vi "ToTable Test.vi"() -> ()   [LabVIEW 2017, in "FPGA Windows Tests.lvlib"]
doc: "Tests the 'To Table' method."
uses:
  FPGA Windows Tests.lvlib
  <vilib>/NI/Module Execution Interface/Engine Configuration/engine configuration.lvclass
  editor node/FPGA Module editor node.lvclass
  <vilib>/NI/Tag Bus/tag/tag descriptor.lvclass
  <vilib>/NI/Tag Bus/tag/Data Type.ctl
  <vilib>/NI/Tag Bus/tag/tag descriptor.lvclass/tag descriptor.ctl
  <vilib>/NI/Configuration Framework/serializable configuration/NISE_CEF_serializable configuration.lvclass/NISE_CEF_serializable configuration.ctl
  module/configuration/FPGA Module configuration.lvclass
  C:/Program Files (x86)/National Instruments/LabVIEW 2017/vi.lib/NI/Configuration Framework/serializable configuration/NISE_CEF_serializable configuration.lvclass
  <vilib>/Utility/LVClass/Get LV Class Name.vi
  <vilib>/NI/Configuration Framework/error generator/NISE_error generator.vi
  <vilib>/NI/Configuration Framework/serializable configuration/NISE_CEF_serializable configuration.lvclass
panel:
  out "error out":errorcluster
  out "table":string[][](array[string])
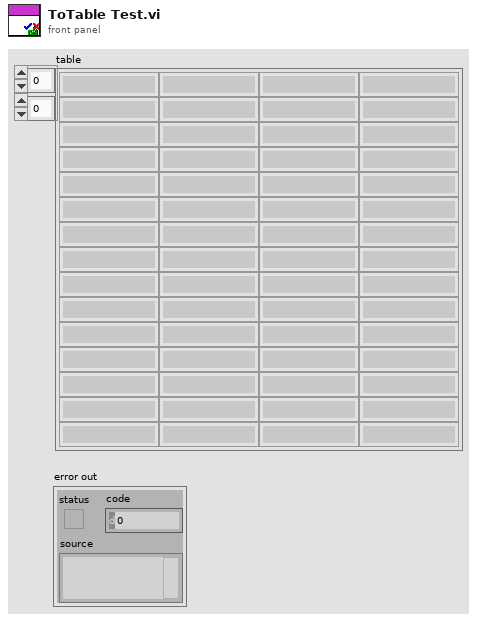
[diagram p1: front panel]
types:
  T1 = typedef "tag bus.lvlib/tag descriptor.lvclass/Data Type.ctl" = enum16{"Double", "Single", "I64", "I32", "I16", "I8", "U64", "U32", "U16", "U8", "Boolean", "String", "Array of Double", "Array of Single", "Array of I64", "Array of I32", "Array of I16", "Array of I8", "Array of U64", "Array of U32", "Array of U16", "Array of U8", "Array of Boolean", "Array of String"}
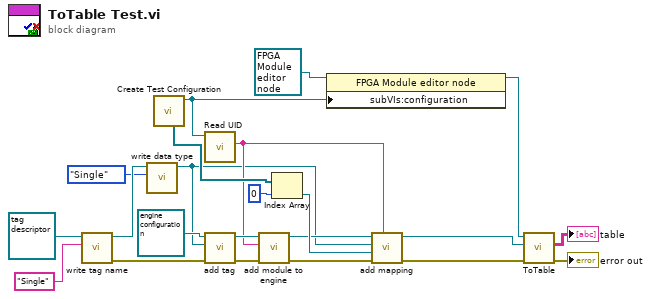
[diagram p0: block diagram]
diagram:
  n1 = call <vilib>:"write tag name.vi"("name"="Single", "system tag in"=refnum<class "tag descriptor.lvclass"> refnum ("tag descriptor")) -> ("error out"=w4:errorcluster, "system tag out"=w3:refnum<class "tag descriptor.lvclass">)  [unwired: 8 in]
  n2 = call <vilib>:"write data type.vi"("data type"=Data_Type."Single", "system tag in"=w3) -> ("system tag out"=w2:refnum<class "tag descriptor.lvclass">)  [unwired: 8 in, 1 out]
  n3 = call "Create Test Configuration.vi"() -> ("Module Configuration"=w12:refnum<class "FPGA Module configuration.lvclass">, "Channels"=w15:refnum<class "TBM channel.lvclass">[])  [unwired: 6 in, 4 out]
  n4 = call <vilib>:"Read UID.vi"("configuration in"=w12) -> ("instance id"=w8:string)  [unwired: 8 in, 2 out]
  n5 = call-dynamic "add tag.vi"("error in"=w4, "tag descriptor"=w2, "engine configuration in"=refnum<class "engine configuration.lvclass"> refnum ("engine configuration")) -> ("error out"=w5:errorcluster, "engine configuration out"=w10:refnum<class "engine configuration.lvclass">)  [unwired: 7 in]
  n6 = call-dynamic "add module to engine.vi"("error in"=w5, "module ID"=w8, "engine configuration in"=w10) -> ("error out"=w7:errorcluster, "engine configuration out"=w9:refnum<class "engine configuration.lvclass">)  [unwired: 7 in]
  n7 = Index Array(array=w15, index=0) -> (element=w13:refnum<class "TBM channel.lvclass">)
  n8 = property class="FPGA Module editor node"(reference=refnum<class "FPGA Module editor node.lvclass"> refnum ("node in"), "subVIs:configuration"=w12) -> (reference out=w21:refnum<class "FPGA Module editor node.lvclass">)  [unwired: 1 in, 1 out]
  n9 = call-dynamic "add mapping.vi"("owner ID"=w8, "error in"=w7, "channel"=w13, "tag descriptor"=w2, "engine configuration"=w9) -> ("error out"=w6:errorcluster, "engine configuration out"=w11:refnum<class "engine configuration.lvclass">)  [unwired: 5 in]
  n10 = call-dynamic "ToTable.vi"("error in"=w6, "variant"=w11, "FPGA Module editor node in"=w21) -> ("error out"=→"error out":errorcluster, "table"=→"table":string[][])  [unwired: 5 in, 2 out]
